vi "arrayTool.vi"(3 "Max Size":i32=100, 4 "New Element":dbl, 5 "Reset?":bool) -> (1 "Array Out":dbl[](array[numeric]))   [LabVIEW 2025]
panel:
  out "queue name":string
  out "created new?":bool
  out "error out":errorcluster
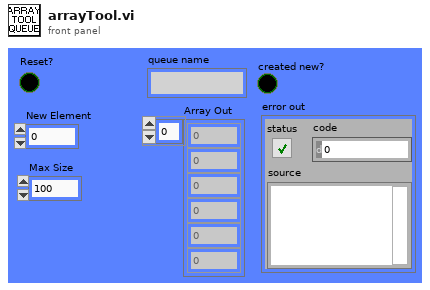
[diagram p1: front panel]
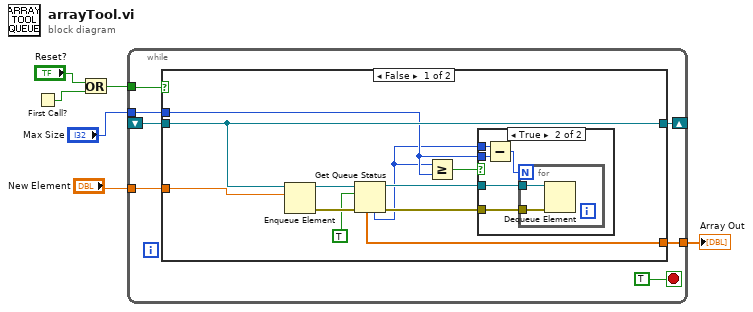
[diagram p0: block diagram]
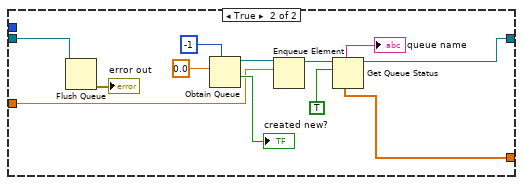
[diagram p3: hidden frame]
diagram:
  n1 = First Call?() -> (First Call?: T/F=w2:bool)
  n2 = Or(x="Reset?", y=w2) -> (x .or. y?=w6:bool)
  n3 = while {
    tunnel: w6 -> [w12]
    shift-right: [w11] -> _
    shift-left: _ -> [w10]
    tunnel: [w9] -> w5
    tunnel: "New Element" -> [w8]
    tunnel: "Max Size" -> [w7]
    stop <- TRUE stop-if-true
    n4 = case shown="False" w12 {
      tunnel: [w24 w36] -> w11
      tunnel: w10 -> [w24 w43]
      tunnel: [w20 w35] -> w9
      tunnel: w8 -> [w16 w38]
      tunnel: w7 -> [w15 _]
      frame False {
        n5 = Enqueue Element(queue=w24, element=w16) -> (queue out=w23:refnum<queue>, error out=w22:errorcluster)  [unwired: 2 in, 1 out]
        n6 = Get Queue Status(queue=w23, return elements? (F)=TRUE, error in (no error)=w22) -> (queue out=w19:refnum<queue>, error out=w18:errorcluster, # elements in queue=w14:i32, elements=w20:dbl[])  [unwired: 4 out]
        n7 = Greater Or Equal?(x=w14, y=w15) -> (x >= y?=w17:bool)
        n8 = case shown="True" w17 {
          tunnel: w19 -> [_ w28]
          tunnel: w18 -> [_ w29]
          tunnel: w15 -> [_ w26]
          tunnel: w14 -> [_ w25]
          frame False {
          }
          frame True {
            n9 = Subtract(x=w25, y=w26) -> (x-y=w27:i32)
            n10 = for {
              N: w27 -> [_]
              tunnel: w29 -> [w31]
              tunnel: w28 -> [w30]
              n11 = Dequeue Element(queue=w30, error in (no error)=w31) -> ()  [unwired: 1 in, 4 out]
            }
          }
        }
      }
      frame True {
        n12 = Flush Queue(queue=w43) -> (error out=→"error out":errorcluster)  [unwired: 1 in, 2 out]
        n13 = Obtain Queue(max queue size (-1, unlimited)=-1, element data type=0.0) -> (queue out=w39:refnum<queue>, created new?=→"created new?":bool)  [unwired: 3 in, 1 out]
        n14 = Enqueue Element(queue=w39, element=w38) -> (queue out=w37:refnum<queue>)  [unwired: 2 in, 2 out]
        n15 = Get Queue Status(queue=w37, return elements? (F)=TRUE) -> (queue out=w36:refnum<queue>, queue name=→"queue name":string, elements=w35:dbl[])  [unwired: 1 in, 5 out]
      }
    }
  }
  "Array Out" <- w5
